vi "CSTK_Icon_Creator_Dialong_CreateLogo.vi"(0 "Enable":bool=TRUE caption="启用", 5 "error in (no error)":errorcluster caption="错误输入（无错误）") -> (18 "确定":bool, 19 "error out":errorcluster caption="错误输出")   [LabVIEW 2015, in "CSTK_Icon Creator.lvlib"]
doc: "显示标准对话框，提示用户输入用户名、密码等信息。\n--------------------\n\n该Express VI配置如下:\n\n显示给用户的信息:请输入分类文件夹名\n该输入为: \n文本输入框: 分类文件夹名"
uses:
  CSTK_Icon Creator.lvlib
  <vilib>/Utility/sysdir.llb/System Directory Type.ctl
  <vilib>/Utility/cursorutil.llb/Set Cursor (Icon Pict).vi
panel:
  in  "ArrowRight":bool
  in  "ArrowLeft":bool
  in  "ArrowDown":bool
  in  "ArrowUp":bool
  in  "导入图片按钮":bool
  in  "Cancel":bool caption="取消"
  in  "OK2":bool
  out "当前坐标颜色值（RGB）":string caption="RGB颜色值"
  out "当前坐标颜色值（HEX）":string caption="HEX颜色值"
  out "当前像素坐标":string
  in  "全部复位颜色":u32(colorbox)=16777215
  in  "右键单击颜色（背景）":u32(colorbox)=16777215
  in  "左键单击颜色（前景）":u32(colorbox)=8421631
  out "LOGO":u32[][](array[colorbox])=[[16777215, 16777215, 16777215, 16777215, 16777215, 16777215, 16777215, 16777215, 16777215], [16777215, 16777215, 16777215, 16777215, 16777215, 16777215, 16777215, 16777215, 16777215], [16777215, 16777215, 16777215, 16777215, 16777215, 16777215, 16777215, 16777215, 16777215], [16777215, 16777215, 16777215, 16777215, 16777215, 16777215, 16777215, 16777215, 16777215], [16777215, 16777215, 16777215, 16777215, 16777215, 16777215, 16777215, 16777215, 16777215], [16777215, 16777215, 16777215, 16777215, 16777215, 16777215, 16777215, 16777215, 16777215], [16777215, 16777215, 16777215, 16777215, 16777215, 16777215, 16777215, 16777215, 16777215]]
  # "LOGO绘图区"
  # "导入图片仅支持9*7像素图片，超过该像素将会被裁切"
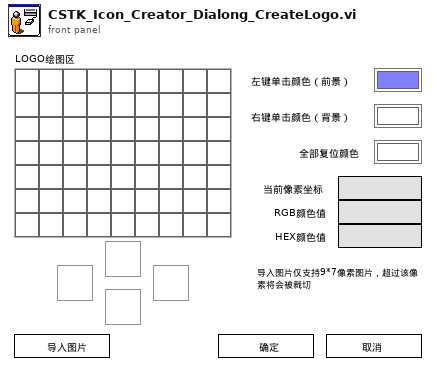
[diagram p1: front panel]
types:
  T1 = typedef "LVPoint32TypeDef.ctl" = cluster{"Horizontal":i32, "Vertical":i32}
  T2 = typedef "System Directory Type.ctl" = i32
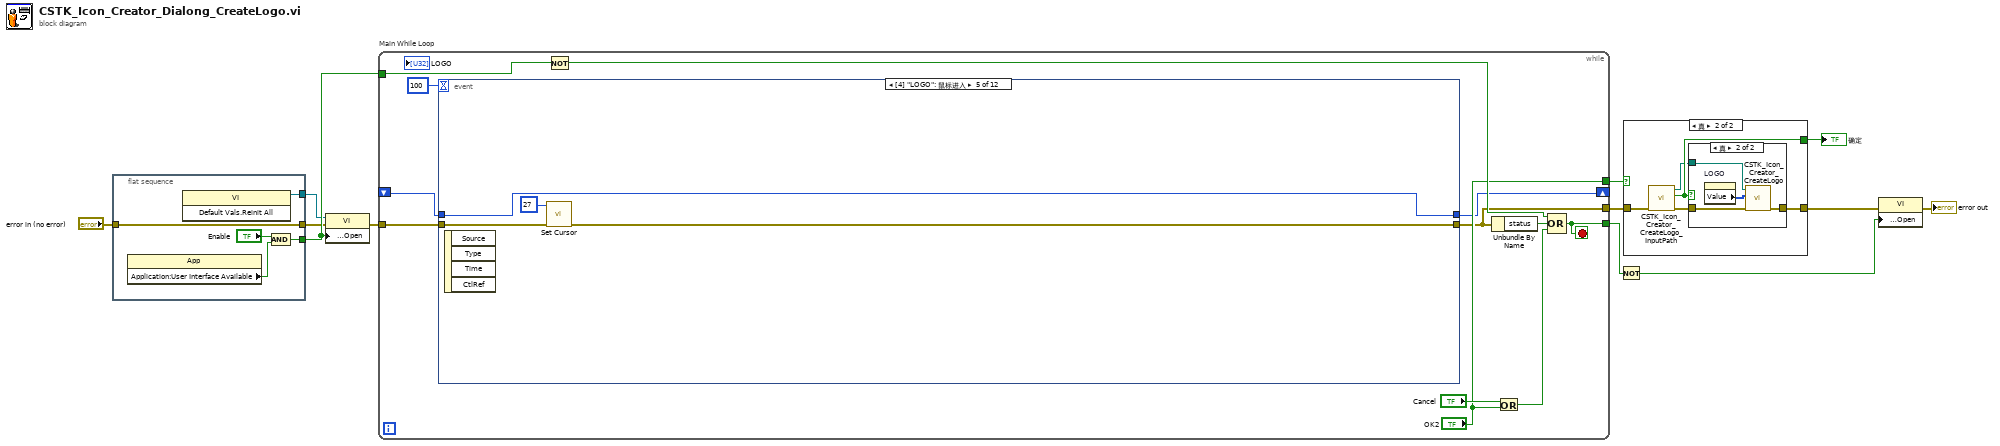
[diagram p0: block diagram]
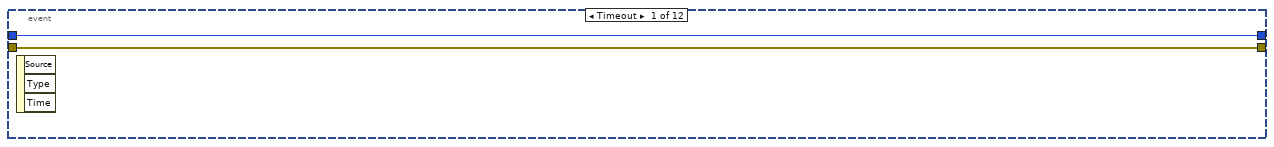
[diagram p4: hidden frame]
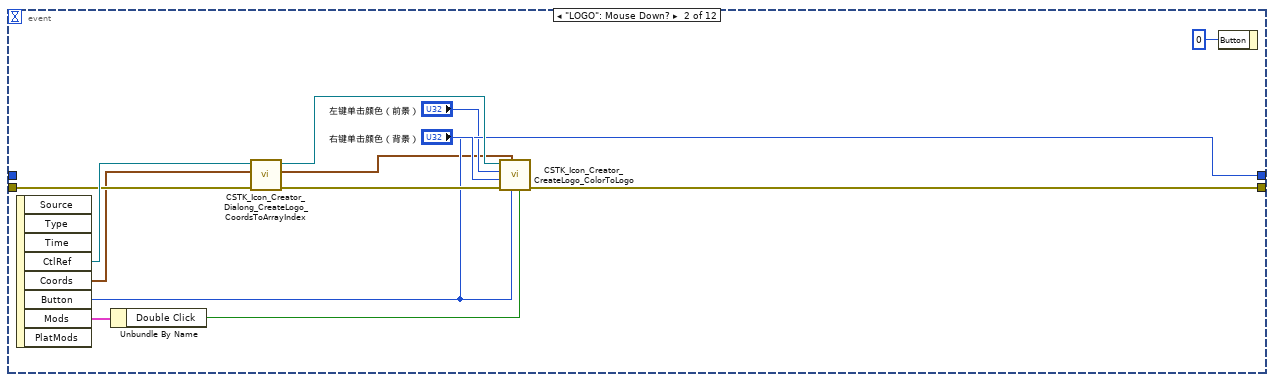
[diagram p5: hidden frame]
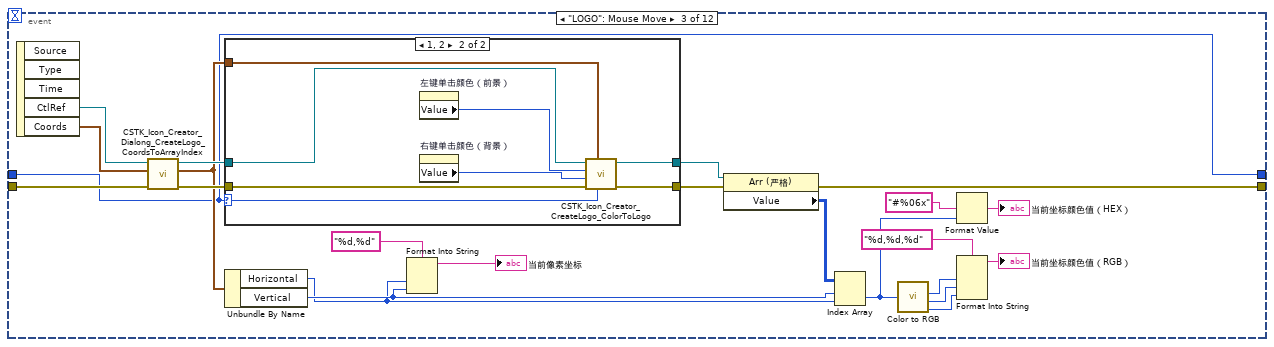
[diagram p6: hidden frame]
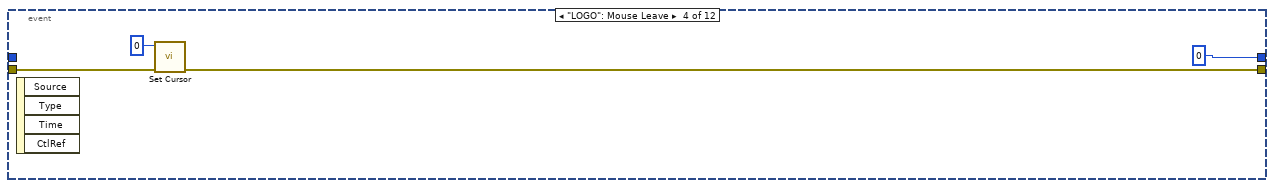
[diagram p8: hidden frame]
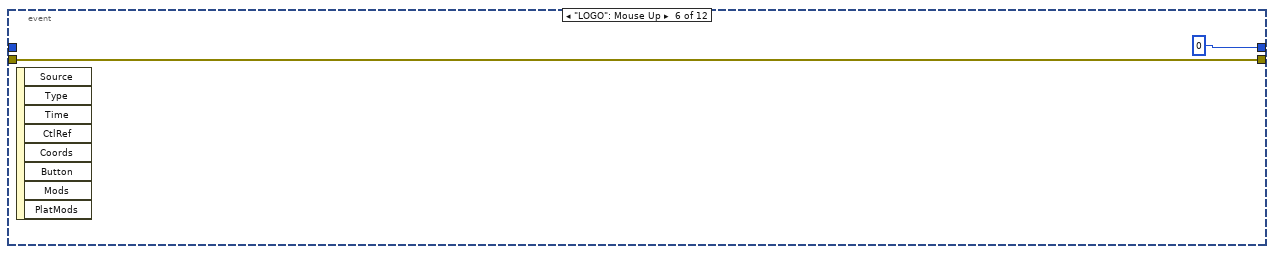
[diagram p9: hidden frame]
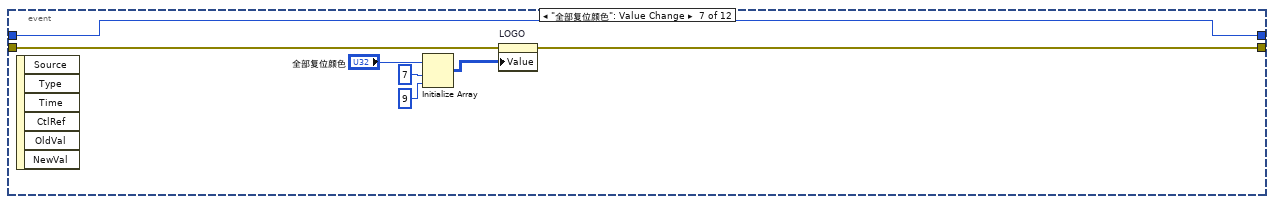
[diagram p10: hidden frame]
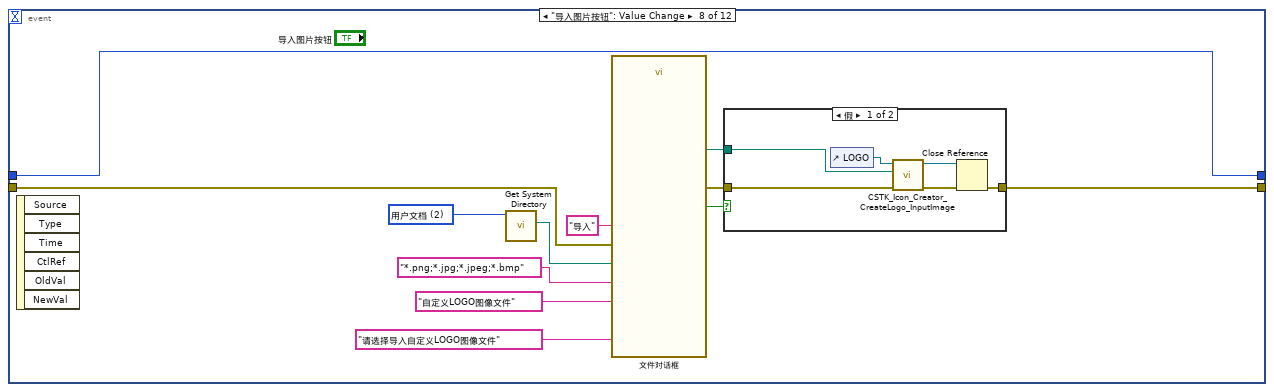
[diagram p11: hidden frame]
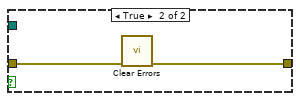
[diagram p12: hidden frame]
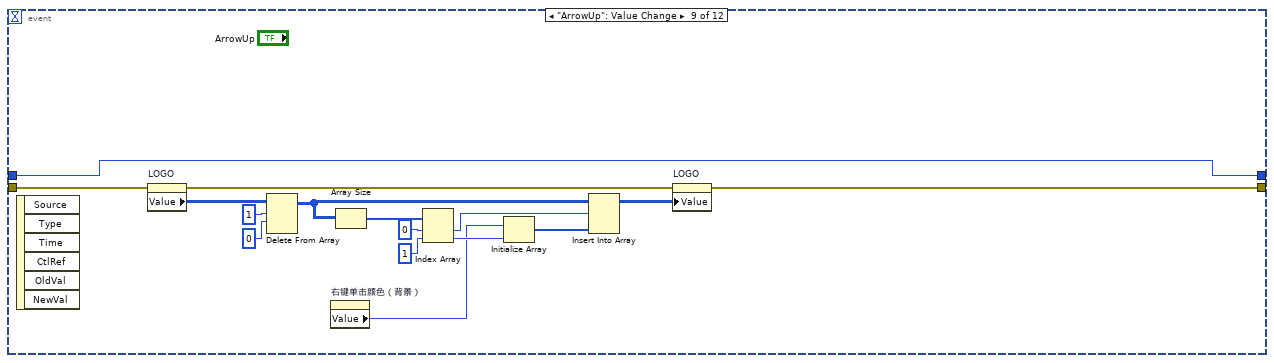
[diagram p13: hidden frame]
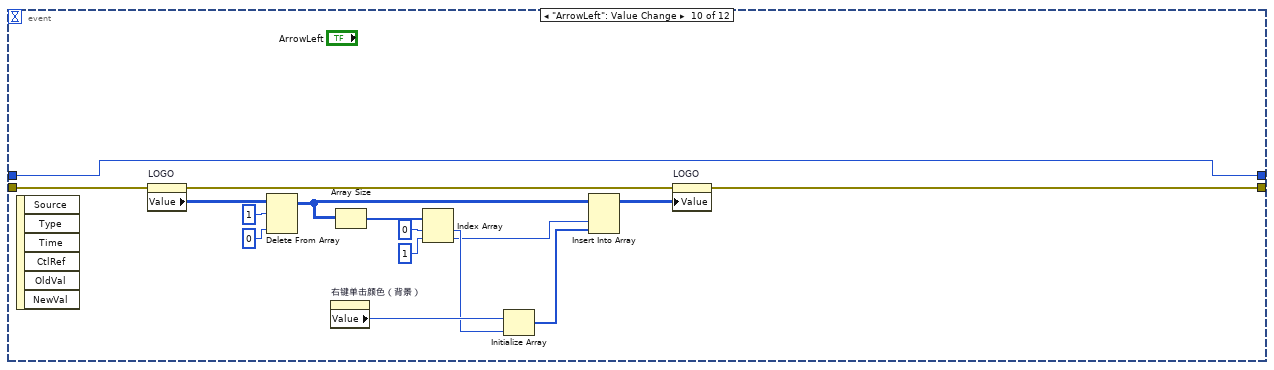
[diagram p14: hidden frame]
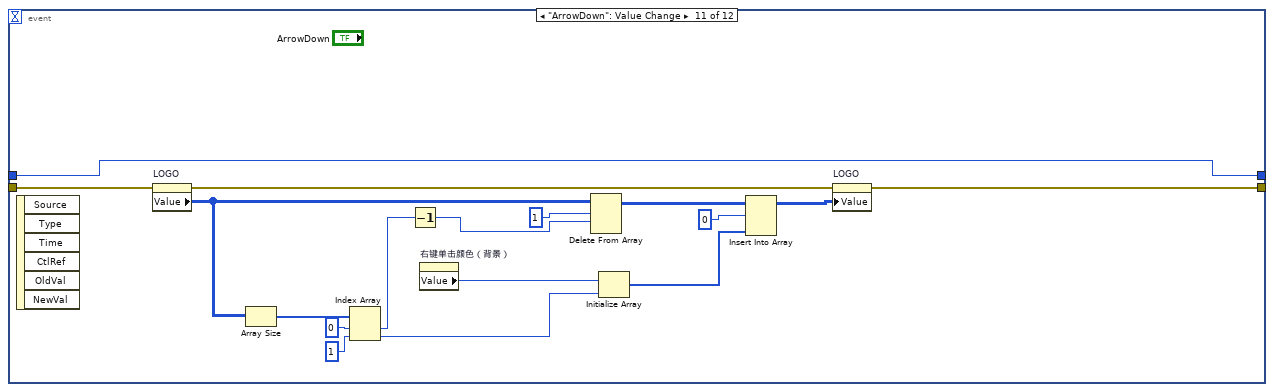
[diagram p15: hidden frame]
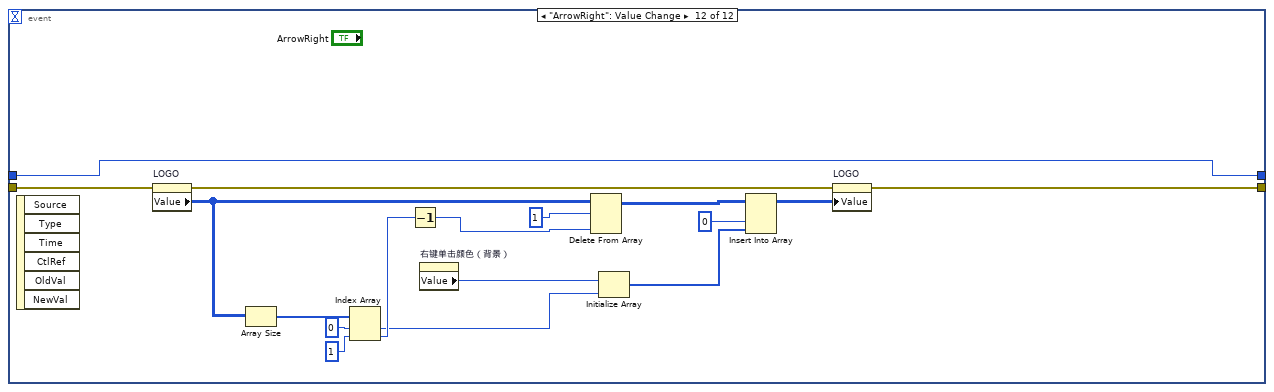
[diagram p16: hidden frame]
diagram:
  n1 = flat-sequence {
    tunnel: [w16] -> w9
    tunnel: [w14] -> w8
    tunnel: [w13] -> w6
    tunnel: "error in (no error)" -> [w13]
    frame #0 {
      n2 = property class="App"() -> ("Application:User Interface Available"=w15:bool)  [unwired: 2 in, 2 out]
      n3 = invoke class="VI" method="Default Vals.Reinit All"() -> (reference out=w14:refnum<vi>)  [unwired: 3 in, 2 out]
      n4 = And(x="Enable", y=w15) -> (x .and. y?=w16:bool)
    }
  }
  n5 = property class="VI"(reference=w8, error in=w6, "Front Panel Window:Open"=w9) -> (error out=w11:errorcluster)  [unwired: 1 out]
  n6 = while "Main While Loop" {
    tunnel: ["OK2"] -> w4
    tunnel: w9 -> [w28]
    tunnel: [w26] -> w12
    tunnel: w11 -> [w21]
    tunnel: [w20] -> w3
    shift-right: [w19] -> _
    shift-left: _ -> [w18]
    stop <- w26 stop-if-true
    n7 = event shown="[4] \"LOGO\": 鼠标进入" {
      selector: _ -> [_ _ _ _ _ _ _ _ _ _ _ _]
      dyn-events: _ -> [_ _ _ _ _ _ _ _ _ _ _ _]
      timeout: u32 100 ("millisecond multiple") -> [_ _ _ _ _ _ _ _ _ _ _ _]
      tunnel: w21 -> [w31 w43 w66 w79 w84 w87 w89 w104 w129 w145 w162 w179]
      tunnel: [w31 w38 w61 w78 w83 w87 w90 w97 w115 w134 w155 w172] -> w20
      tunnel: [w30 w34 w46 u16 0 ("Button") w82 u16 0 ("Button") w88 w106 w130 w146 w163 w180] -> w19
      tunnel: w18 -> [w30 _ w46 _ w82 _ w88 w106 w130 w146 w163 w180]
      event Timeout {
        n8 = event-data() -> ()  [unwired: 1 in, 3 out]
      }
      event "LOGO": Mouse Down? {
        n9 = event-data() -> ("CtlRef"=w44:refnum<vi>, "Coords"=w42:T1, "Button"=w34:u16, "Mods"=w40:cluster{"Double Click":bool, "Menu Key":bool})  [unwired: 1 in, 4 out]
        n10 = Unbundle By Name(w40) -> ("Double Click"=w35:bool)
        n11 = call "CSTK_Icon_Creator_Dialong_CreateLogo_CoordsToArrayIndex.vi"("错误输入（无错误）"=w43, "Coords"=w42, "Array输入"=w44) -> ("错误输出"=w39:errorcluster, "ArrayIndex"=w32:T1, "Array输出"=w36:refnum<vi>)  [unwired: 6 in]
        n12 = call "CSTK_Icon_Creator_CreateLogo_ColorToLogo.vi"("Double Click"=w35, "Button"=w34, "ArrayIndex"=w32, "错误输入（无错误）"=w39, "右键单击颜色"="右键单击颜色（背景）", "左键单击颜色"="左键单击颜色（前景）", "LOGO输入"=w36) -> ("错误输出"=w38:errorcluster)  [unwired: 3 in, 1 out]
        n13 = event-data("Button"=u16 0 ("按钮")) -> ()  [unwired: 1 in, 1 out]
      }
      event "LOGO": Mouse Move {
        n14 = event-data() -> ("CtlRef"=w67:refnum<vi>, "Coords"=w65:T1)  [unwired: 1 in, 3 out]
        n15 = call "CSTK_Icon_Creator_Dialong_CreateLogo_CoordsToArrayIndex.vi"("错误输入（无错误）"=w66, "Coords"=w65, "Array输入"=w67) -> ("错误输出"=w50:errorcluster, "ArrayIndex"=w47:T1, "Array输出"=w48:refnum<vi>)  [unwired: 6 in]
        n16 = case shown="1, 2" w46 {
          selector: w46 -> [_ w70]
          tunnel: w50 -> [w69 w77]
          tunnel: [w69 w76] -> w49
          tunnel: w48 -> [w68 w75]
          tunnel: w47 -> [_ w74]
          tunnel: [w68 w71] -> w45
          frame Default {
          }
          frame 1, 2 {
            n17 = property on="左键单击颜色（前景）" class="ColBox"() -> ("Value"=w73:u32)  [unwired: 2 in, 2 out]
            n18 = property on="右键单击颜色（背景）" class="ColBox"() -> ("Value"=w72:u32)  [unwired: 2 in, 2 out]
            n19 = call "CSTK_Icon_Creator_CreateLogo_ColorToLogo.vi"("Button"=w70, "ArrayIndex"=w74, "错误输入（无错误）"=w77, "右键单击颜色"=w72, "左键单击颜色"=w73, "LOGO输入"=w75) -> ("错误输出"=w76:errorcluster, "LOGO输出"=w71:refnum<vi>)  [unwired: 4 in]
          }
        }
        n20 = Unbundle By Name(w47) -> ("Horizontal"=w51:i32, "Vertical"=w52:i32)
        n21 = Format Into String(format string="%d,%d" ("格式字符串"), w51, w52) -> (resulting string=→"当前像素坐标":string)  [unwired: 2 in, 1 out]
        n22 = property on="属性节点" class="Arr (严格)"(reference=w45, error in=w49) -> (error out=w61:errorcluster, "Value"=w62:u32[][])  [unwired: 1 out]
        n23 = Index Array(array=w62, index (row)=w52, index (col)=w51) -> (element=w58:u32)
        n24 = call <vilib>:"Color to RGB.vi"("Color"=w58) -> ("R"=w56:u8, "G"=w55:u8, "B"=w54:u8)  [unwired: 1 out]
        n25 = Format Value(format string="#%06x" ("格式字符串"), value (0)=w58) -> (output string=→"当前坐标颜色值（HEX）":string)  [unwired: 1 in]
        n26 = Format Into String(format string="%d,%d,%d" ("格式字符串"), w56, w55, w54) -> (resulting string=→"当前坐标颜色值（RGB）":string)  [unwired: 2 in, 1 out]
      }
      event "LOGO": Mouse Leave {
        n27 = event-data() -> ()  [unwired: 1 in, 4 out]
        n28 = call-poly <vilib>:"Set Cursor.vi"("error in (no error)"=w79, "icon"=u16 0) -> ("error out"=w78:errorcluster)  [unwired: 8 in, 1 out]
      }
      event "LOGO": Mouse Enter {
        n29 = event-data() -> ()  [unwired: 1 in, 4 out]
        n30 = call-poly <vilib>:"Set Cursor.vi"("error in (no error)"=w84, "icon"=u16 27) -> ("error out"=w83:errorcluster)  [unwired: 8 in, 1 out]
      }
      event "LOGO": Mouse Up {
        n31 = event-data() -> ()  [unwired: 1 in, 8 out]
      }
      event "全部复位颜色": Value Change {
        n32 = event-data() -> ()  [unwired: 1 in, 6 out]
        n33 = Initialize Array("全部复位颜色", 7 ("维数大小"), 9 ("维数大小")) -> (w91:u32[][])
        n34 = property on="LOGO" class="Arr (严格)"(error in=w89, "Value"=w91) -> (error out=w90:errorcluster)  [unwired: 1 in, 1 out]
      }
      event "导入图片按钮": Value Change {
        w103 = T2 2 items=["用户目录"=0, "用户桌面"=1, "用户文档"=2, "用户应用程序数据"=3, "用户设置"=4, "用户临时目录"=5, "公共文档"=6, "公共应用程序数据"=7, "公共设置"=8, "公共缓存"=13, "系统核心库"=9, "系统安装库"=10, "应用程序文件"=11, "启动盘根目录"=12] ("system directory type")
        n35 = event-data() -> ()  [unwired: 1 in, 6 out]
        n36 = call <vilib>:"Get System Directory.vi"("system directory type"=w103) -> ("system directory"=w102:path)  [unwired: 10 in]
        n37 = call "文件对话框"("start path"=w102, "prompt"="请选择导入自定义LOGO图像文件" ("default name"), "button label"="导入", "error in"=w104, "pattern (all files)"="*.png;*.jpg;*.jpeg;*.bmp", "pattern label"="自定义LOGO图像文件") -> ("selected path"=w95:path, "cancelled"=w98:bool, "error out"=w96:errorcluster)  [unwired: 6 in, 1 out]
        n38 = case shown="假" w98 {
          tunnel: [w107 w113] -> w97
          tunnel: w96 -> [w111 w114]
          tunnel: w95 -> [w112 _]
          frame False {
            n39 = control-ref of="LOGO"() -> (w110:refnum<vi>)
            n40 = call "CSTK_Icon_Creator_CreateLogo_InputImage.vi"("错误输入（无错误）"=w111, "LOGO图像路径"=w112, "LOGO输入"=w110) -> ("错误输出"=w109:errorcluster, "LOGO输出"=w108:refnum<vi>)  [unwired: 7 in]
            n41 = Close Reference(reference=w108, error in (no error)=w109) -> (error out=w107:errorcluster)
          }
          frame True {
            n42 = call <vilib>:"Clear Errors.vi"("error in (no error)"=w114) -> ("error out"=w113:errorcluster)  [unwired: 5 in, 1 out]
          }
        }
      }
      event "ArrowUp": Value Change {
        n43 = event-data() -> ()  [unwired: 1 in, 6 out]
        n44 = property on="LOGO" class="Arr (严格)"(error in=w129) -> (error out=w116:errorcluster, "Value"=w128:u32[][])  [unwired: 1 in, 1 out]
        n45 = Delete From Array(array=w128, length=1 ("长度"), index (row)=0 ("索引 (行)")) -> (array with subset deleted=w125:u32[][])  [unwired: 1 in, 1 out]
        n46 = property on="右键单击颜色（背景）" class="ColBox"() -> ("Value"=w119:u32)  [unwired: 2 in, 2 out]
        n47 = Array Size(array=w125) -> (size(s)=w124:i32[])
        n48 = Index Array(array=w124, index #1=0 ("索引"), index #2=1 ("索引")) -> (element #1=w122:i32, element #2=w120:i32)
        n49 = Initialize Array(w119, w120) -> (w118:u32[])
        n50 = Insert Into Array(array=w125, index (row)=w122, new element=w118) -> (w117:u32[][])  [unwired: 1 in]
        n51 = property on="LOGO" class="Arr (严格)"(error in=w116, "Value"=w117) -> (error out=w115:errorcluster)  [unwired: 1 in, 1 out]
      }
      event "ArrowLeft": Value Change {
        n52 = event-data() -> ()  [unwired: 1 in, 6 out]
        n53 = property on="LOGO" class="Arr (严格)"(error in=w145) -> (error out=w135:errorcluster, "Value"=w144:u32[][])  [unwired: 1 in, 1 out]
        n54 = Delete From Array(array=w144, length=1 ("长度"), index (col)=0 ("索引 (行)")) -> (array with subset deleted=w142:u32[][])  [unwired: 1 in, 1 out]
        n55 = property on="右键单击颜色（背景）" class="ColBox"() -> ("Value"=w138:u32)  [unwired: 2 in, 2 out]
        n56 = Array Size(array=w142) -> (size(s)=w141:i32[])
        n57 = Index Array(array=w141, index #1=0 ("索引"), index #2=1 ("索引")) -> (element #1=w132:i32, element #2=w131:i32)
        n58 = Initialize Array(w138, w132) -> (w137:u32[])
        n59 = Insert Into Array(array=w142, index (col)=w131, new element=w137) -> (w136:u32[][])  [unwired: 1 in]
        n60 = property on="LOGO" class="Arr (严格)"(error in=w135, "Value"=w136) -> (error out=w134:errorcluster)  [unwired: 1 in, 1 out]
      }
      event "ArrowDown": Value Change {
        n61 = event-data() -> ()  [unwired: 1 in, 6 out]
        n62 = property on="LOGO" class="Arr (严格)"(error in=w162) -> (error out=w156:errorcluster, "Value"=w154:u32[][])  [unwired: 1 in, 1 out]
        n63 = Array Size(array=w154) -> (size(s)=w151:i32[])
        n64 = Index Array(array=w151, index #1=0 ("索引"), index #2=1 ("索引")) -> (element #1=w150:i32, element #2=w147:i32)
        n65 = Decrement(x=w150) -> (x-1=w149:i32)
        n66 = property on="右键单击颜色（背景）" class="ColBox"() -> ("Value"=w159:u32)  [unwired: 2 in, 2 out]
        n67 = Delete From Array(array=w154, length=1 ("长度"), index (row)=w149) -> (array with subset deleted=w160:u32[][])  [unwired: 1 in, 1 out]
        n68 = Initialize Array(w159, w147) -> (w158:u32[])
        n69 = Insert Into Array(array=w160, index (row)=0 ("索引"), new element=w158) -> (w157:u32[][])  [unwired: 1 in]
        n70 = property on="LOGO" class="Arr (严格)"(error in=w156, "Value"=w157) -> (error out=w155:errorcluster)  [unwired: 1 in, 1 out]
      }
      event "ArrowRight": Value Change {
        n71 = event-data() -> ()  [unwired: 1 in, 6 out]
        n72 = property on="LOGO" class="Arr (严格)"(error in=w179) -> (error out=w173:errorcluster, "Value"=w171:u32[][])  [unwired: 1 in, 1 out]
        n73 = Array Size(array=w171) -> (size(s)=w168:i32[])
        n74 = Index Array(array=w168, index #1=0 ("索引"), index #2=1 ("索引")) -> (element #1=w165:i32, element #2=w167:i32)
        n75 = Decrement(x=w167) -> (x-1=w166:i32)
        n76 = property on="右键单击颜色（背景）" class="ColBox"() -> ("Value"=w176:u32)  [unwired: 2 in, 2 out]
        n77 = Delete From Array(array=w171, length=1 ("长度"), index (col)=w166) -> (array with subset deleted=w177:u32[][])  [unwired: 1 in, 1 out]
        n78 = Initialize Array(w176, w165) -> (w175:u32[])
        n79 = Insert Into Array(array=w177, index (col)=0 ("索引"), new element=w175) -> (w174:u32[][])  [unwired: 1 in]
        n80 = property on="LOGO" class="Arr (严格)"(error in=w173, "Value"=w174) -> (error out=w172:errorcluster)  [unwired: 1 in, 1 out]
      }
    }
    n81 = Not(x=w28) -> (.not. x?=w27:bool)
    n82 = Unbundle By Name(w20) -> ("status"=w24:bool)
    n83 = Or(x="Cancel", y="OK2") -> (x .or. y?=w25:bool)
    n84 = Compound Arithmetic op=OR(w27, w24, w25) -> (w26:bool)
  }
  n85 = Not(x=w12) -> (.not. x?=w5:bool)
  n86 = case shown="真" w4 {
    selector: w4 -> [w181 _]
    tunnel: [w182 w183] -> w2
    tunnel: w3 -> [w182 w187]
    tunnel: [w181 w186] -> w1
    frame False {
    }
    frame True {
      n87 = call "CSTK_Icon_Creator_CreateLogo_InputPath.vi"("错误输入（无错误）"=w187) -> ("错误输出"=w184:errorcluster, "OK?"=w186:bool, "文件夹路径输出"=w185:path)  [unwired: 8 in]
      n88 = case shown="真" w186 {
        tunnel: w185 -> [_ w192]
        tunnel: [w188 w189] -> w183
        tunnel: w184 -> [w188 w191]
        frame False {
        }
        frame True {
          n89 = property on="LOGO" class="Arr (严格)"() -> ("Value"=w190:u32[][])  [unwired: 2 in, 2 out]
          n90 = call "CSTK_Icon_Creator_CreateLogo.vi"("错误输入（无错误）"=w191, "LOGO输入"=w190, "文件夹路径输入"=w192) -> ("错误输出"=w189:errorcluster)  [unwired: 8 in]
        }
      }
    }
  }
  "确定" <- w1
  n91 = property class="VI"(error in=w2, "Front Panel Window:Open"=w5) -> (error out=→"error out":errorcluster)  [unwired: 1 in, 1 out]
